vi "DefaultFromIni.vi"(8 "error in (no error)":errorcluster, 11 "SyncPlugin":refnum<class "Local.lvclass">) -> (0 "error out":errorcluster, 3 "SyncPlugin":refnum<class "Local.lvclass">)   [LabVIEW 2014, in "SyncPlugins.lvlib" / "Local.lvclass"]
uses:
  Local.lvclass
  SyncPluginBase/SyncPluginBase.lvclass
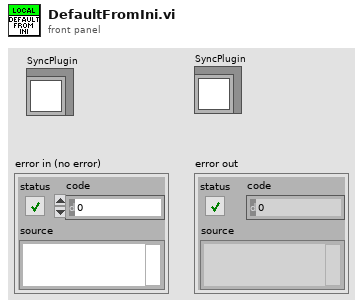
[diagram p1: front panel]
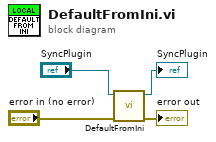
[diagram p0: block diagram]
diagram:
  n1 = call-parent "DefaultFromIni.vi"("error in (no error)"="error in (no error)", "SyncPlugin"="SyncPlugin") -> ("error out"=→"error out":errorcluster, "SyncPlugin"=→"SyncPlugin":refnum<class "Local.lvclass">)  [unwired: 8 in]
